vi "sub_depacket.vi"(10 "bitstream":i8[](array[numeric])) -> (2 "frame":cluster{u32, "string":string})   [LabVIEW 2014]
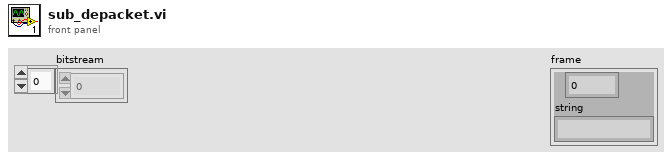
[diagram p1: front panel]
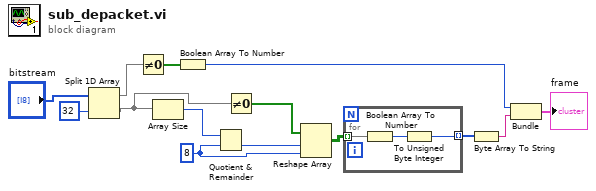
[diagram p0: block diagram]
diagram:
  w12 = 8 ("y")
  n1 = Split 1D Array(array="bitstream", index=32) -> (first subarray=w6:i8[], second subarray=w8:i8[])
  n2 = Not Equal To 0?(x=w6) -> (x != 0?=w5:bool[])
  n3 = Array Size(array=w8) -> (size(s)=w14:i32)
  n4 = Boolean Array To Number(Boolean array=w5) -> (number=w2:u32)
  n5 = Quotient & Remainder(x=w14, y=w12) -> (floor(x/y)=w11:i32)  [unwired: 1 out]
  n6 = Not Equal To 0?(x=w8) -> (x != 0?=w13:bool[])
  n7 = Reshape Array(w13, w11, w12) -> (w10:bool[][])
  n8 = for {
    tunnel: [w17] -> w4 mode=indexing
    tunnel: w10 -> [w15] mode=indexing
    n9 = Boolean Array To Number(Boolean array=w15) -> (number=w16:u32)
    n10 = To Unsigned Byte Integer(number=w16) -> (unsigned 8bit integer=w17:u8)
  }
  n11 = Byte Array To String(unsigned byte array=w4) -> (string=w3:string)
  n12 = Bundle(w2, "string"=w3) -> (→"frame":cluster{u32, "string":string})  [unwired: 1 in]
